vi "Test.vi"() -> ()   [LabVIEW 2022 SP3, in "TimingControl.lvlib" / "TimingControl.lvclass"]
uses:
  TimingControl.lvclass
panel:
  in  "仪器状态":bool
  out "数据":cluster{"启动":bool, "控制命令":T1, "测量参数":T2}
  in  "布尔":bool
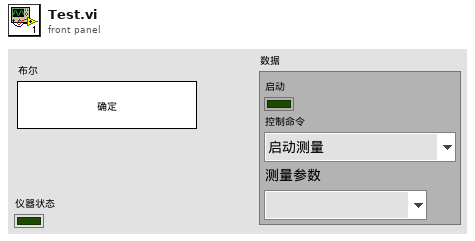
[diagram p1: front panel]
types:
  T1 = typedef "TimingControl.lvlib/TimingControl.lvclass/国标控制命令.ctl" = enum16{"启动测量", "标样核查", "零点核查", "跨度核查", "空白测试", "平行样测试", "加标回收", "空白校准", "标样校准", "初始化（清洗）", "停止测试", "仪器重启", "校时", "模式设置", "测量间隔设置"}
  T2 = typedef "TimingControl.lvlib/TimingControl.lvclass/测量参数.ctl" = u16
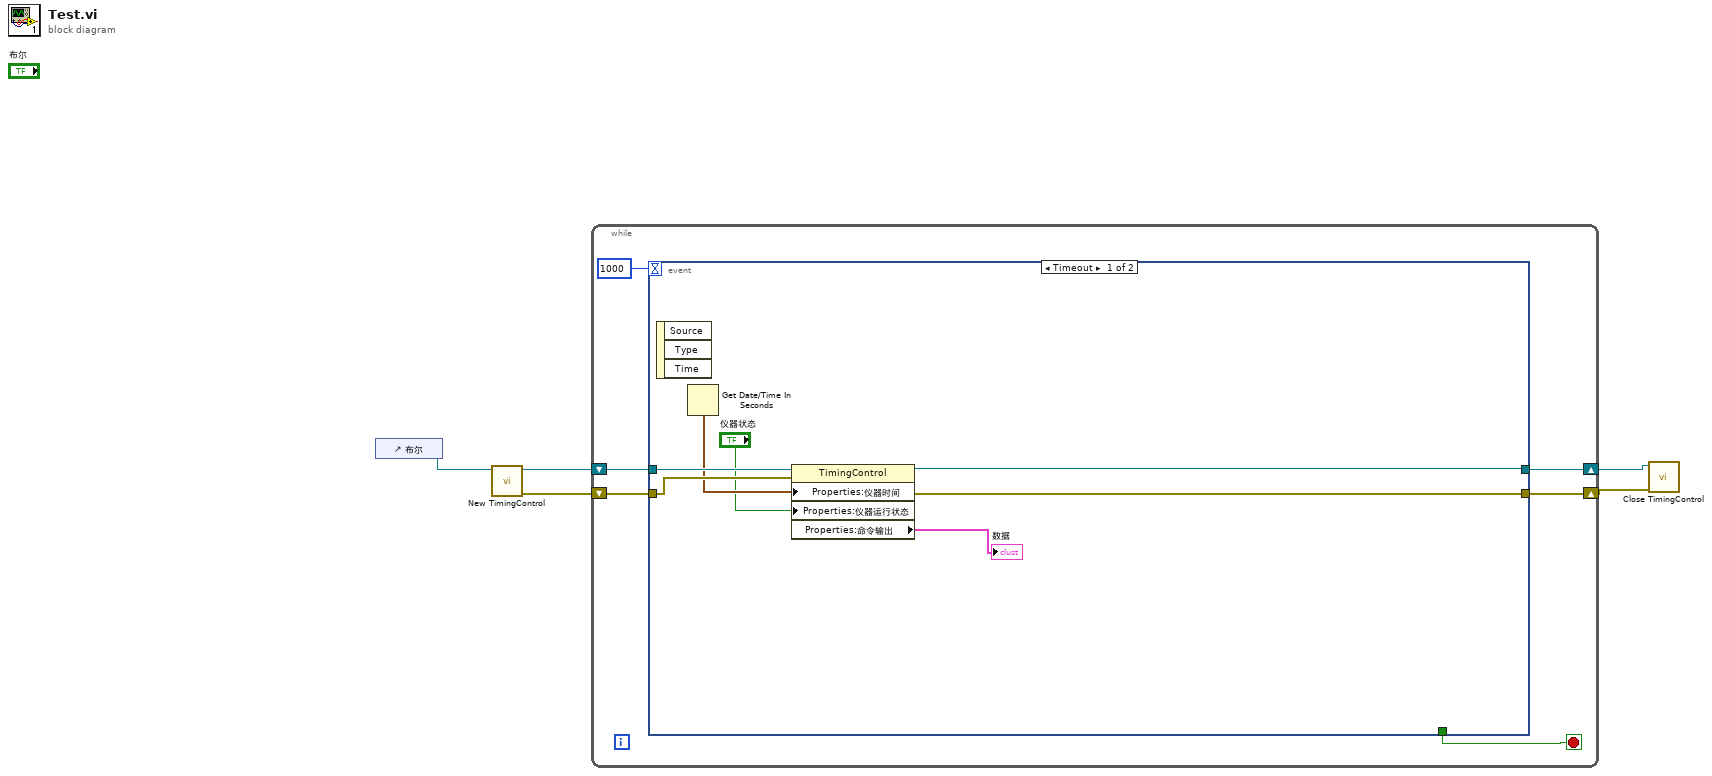
[diagram p0: block diagram]
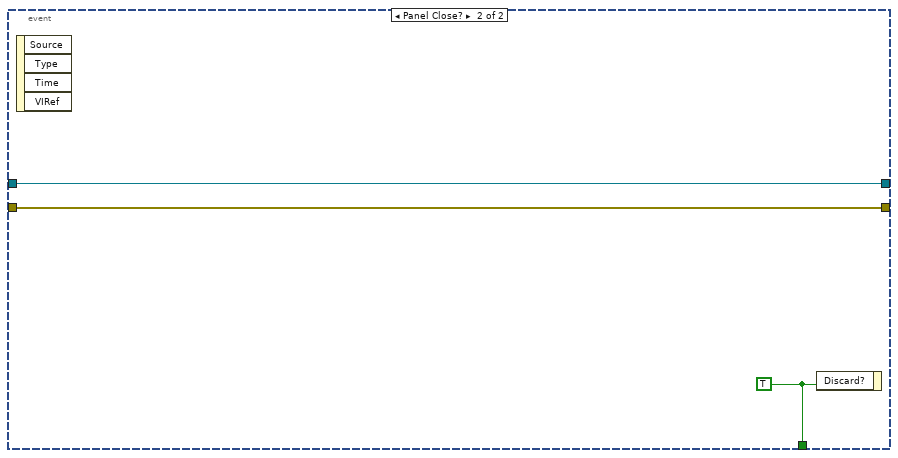
[diagram p2: hidden frame]
diagram:
  n1 = control-ref of="布尔"() -> (w5:refnum<vi>)
  n2 = call "New TimingControl.vi"("Reference"=w5) -> ("error out"=w3:errorcluster, "TimingControl out"=w4:refnum<class "TimingControl.lvclass">)  [unwired: 9 in]
  n3 = while {
    shift-right: [w8] -> w2
    shift-left: w4 -> [w10]
    shift-right: [w7] -> w1
    shift-left: w3 -> [w9]
    stop <- w11 stop-if-true
    n4 = event shown="[0] Timeout" {
      selector: _ -> [_ _]
      dyn-events: _ -> [_ _]
      timeout: 1000 -> [_ _]
      tunnel: [_ w21] -> w11
      tunnel: w10 -> [w15 w20]
      tunnel: w9 -> [w16 w19]
      tunnel: [w18 w20] -> w8
      tunnel: [w17 w19] -> w7
      event Timeout {
        n5 = event-data() -> ()  [unwired: 1 in, 3 out]
        n6 = Get Date/Time In Seconds() -> (seconds since 1Jan1904=w14:timestamp)
        n7 = property class="TimingControl"(reference=w15, error in=w16, "Properties:仪器时间"=w14, "Properties:仪器运行状态"="仪器状态") -> (reference out=w18:refnum<class "TimingControl.lvclass">, error out=w17:errorcluster, "Properties:命令输出"=→"数据":cluster{"启动":bool, "控制命令":T1, "测量参数":T2})
      }
      event Panel Close? {
        w21 = TRUE
        n8 = event-data() -> ()  [unwired: 1 in, 4 out]
        n9 = event-data("Discard?"=w21) -> ()  [unwired: 1 in, 1 out]
      }
    }
  }
  n10 = call "Close TimingControl.vi"("error in (no error)"=w1, "TimingControl in"=w2) -> ()  [unwired: 9 in, 1 out]
